vi "Get Parameter.vi"(8 "error in (no error)":errorcluster, 10 "Name":string, 11 "id":i32) -> (0 "error out":errorcluster, 1 "found?":bool, 3 "value":string)   [LabVIEW 2020, in "MCP Server.lvlib"]
doc: "Returns a parameter passed along with the mcp calls. These parameters can be specified freely with name+value in the mcp_config.json file. Use parameters for user-specific information, api-keys, login information etc."
uses:
  MCP Server.lvlib
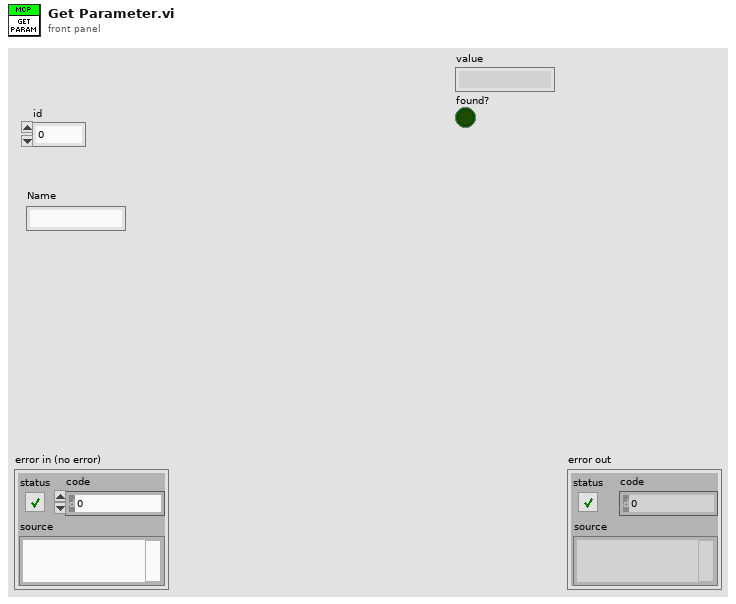
[diagram p1: front panel]
types:
  T1 = typedef "MCP Server.lvlib/Server Data.ctl" = cluster{"Name":string, "Description":string, "Tools":T2[], "Parameters":string[][], "Logging Info":T5, "User Events":T6, "Prompts":T7[], "resources":T9[], "HTTP Server":refnum<class "Server.lvclass">}
  T2 = typedef "MCP Server.lvlib/Tool Data.ctl" = cluster{"Name":string, "Description":string, "Ignored":string[], "inputs":T3[], "outputs":T4[], "VI Refnum":refnum<vi>}
  T3 = typedef "MCP Server.lvlib/Input Parameter.ctl" = cluster{"name":string, "type":string, "description":string, "required":bool, "raw name":string}
  T4 = typedef "MCP Server.lvlib/Output Parameter.ctl" = cluster{"name":string, "description":string, "type":string, "raw name":string}
  T5 = typedef "MCP Server.lvlib/Logging.ctl" = cluster{"Log":string[], "Max Length":i32}
  T6 = typedef "MCP Server.lvlib/User Events.ctl" = cluster{"onError":refnum<user-event>, "onRpc":refnum<user-event>}
  T7 = typedef "MCP Server.lvlib/Prompt Data.ctl" = cluster{"name":string, "description":string, "arguments":T8[], "return terminal name":string, "results description":string, "VI Refnum":refnum<vi>}
  T8 = typedef "MCP Server.lvlib/Prompt Argument.ctl" = cluster{"name":string, "description":string, "required":bool, "raw_name":string}
  T9 = typedef "MCP Server.lvlib/resource data.ctl" = cluster{"uri":string, "name":string, "description":string, "mimeType":string, "file path":path}
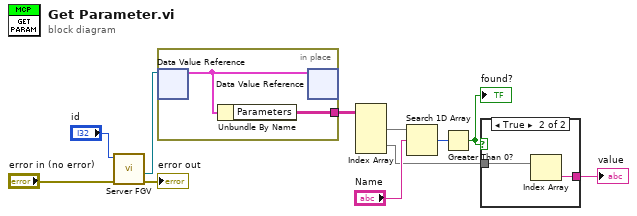
[diagram p0: block diagram]
diagram:
  n1 = call "Server FGV.vi"("error in"="error in (no error)", "id"="id") -> ("error out"=→"error out":errorcluster, "server reference"=w8:refnum<data-value>)  [unwired: 5 in, 3 out]
  n2 = in-place {
    in-place-border: [w12] -> w3
    n3 = in-place-dvr #1(w8) -> (w13:T1)  [unwired: 1 out]
    n4 = Unbundle By Name(w13) -> ("Parameters"=w12:string[][])
    n5 = in-place-dvr #1(w13) -> ()  [unwired: 2 out]
  }
  n6 = Index Array(array=w3) -> (element #1=w7:string[], element #2=w2:string[])  [unwired: 4 in]
  n7 = Search 1D Array(1D array=w7, element="Name") -> (index of element=w5:i32)  [unwired: 1 in]
  n8 = Greater Than 0?(x=w5) -> (x > 0?=w4:bool)
  "found?" <- w4
  n9 = case shown="True" w4 {
    tunnel: w2 -> [_ w15]
    tunnel: [_ w14] -> w1
    frame False {
    }
    frame True {
      n10 = Index Array(array=w15) -> (element=w14:string)  [unwired: 1 in]
    }
  }
  "value" <- w1
